vi "Tri. Flow Model (SubVI).vi"(6 "Offset":dbl, 7 "T_Flow Start (s)":dbl, 8 "T_Ejection Period (s)":dbl, 9 "Pressure (mmHg)":waveform(dbl), 10 "T_Flow Peak (s)":dbl, 11 "Flow Amp.":dbl) -> (3 "Triangular  Model Flow":waveform(dbl))   [LabVIEW 2017]
uses:
  <vilib>/Analysis/NI_AALBase.lvlib
  <vilib>/Analysis/1siggen.llb/Ramp Pattern by Samples.vi
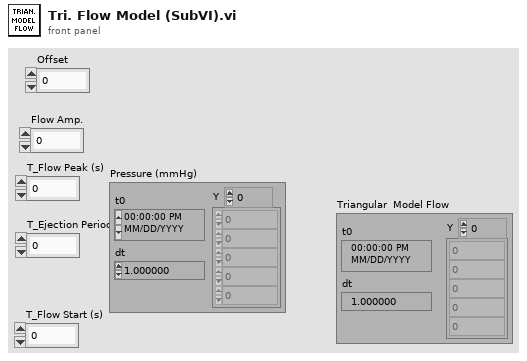
[diagram p1: front panel]
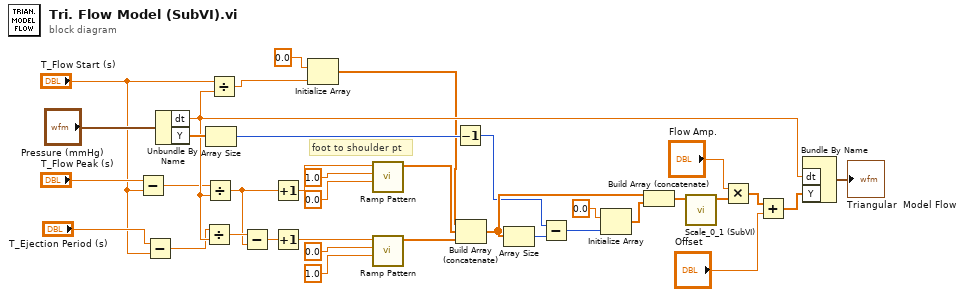
[diagram p0: block diagram]
diagram:
  # "foot to shoulder pt"
  n1 = Subtract(x="T_Flow Peak (s)", y="T_Flow Start (s)") -> (x-y=w4:dbl)
  n2 = Subtract(x="T_Ejection Period (s)", y="T_Flow Start (s)") -> (x-y=w1:dbl)
  n3 = Unbundle By Name("Pressure (mmHg)") -> ("dt"=w13:dbl, "Y"=w17:dbl[])
  n4 = Divide(x=w1, y=w13) -> (x/y=w36:dbl)
  n5 = Divide(x=w4, y=w13) -> (x/y=w21:dbl)
  n6 = Array Size(array=w17) -> (size(s)=w22:i32)
  n7 = Divide(x="T_Flow Start (s)", y=w13) -> (x/y=w10:dbl)
  n8 = Subtract(x=w36, y=w21) -> (x-y=w34:dbl)
  n9 = Increment(x=w21) -> (x+1=w33:dbl)
  n10 = Increment(x=w34) -> (x+1=w35:dbl)
  n11 = Initialize Array(0.0 ("element"), w10) -> (w11:dbl[])
  n12 = call-poly <vilib>:"Ramp Pattern.vi"("start"=0.0, "end"=1.0, "samples"=w33) -> ("Ramp Pattern"=w32:dbl[])  [unwired: 7 in, 1 out]
  n13 = call-poly <vilib>:"Ramp Pattern.vi"("start"=1.0, "end"=0.0, "samples"=w35) -> ("Ramp Pattern"=w20:dbl[])  [unwired: 7 in, 1 out]
  n14 = Decrement(x=w22) -> (x-1=w19:i32)
  n15 = Build Array (concatenate)(w11, w32, w20) -> (w23:dbl[])
  n16 = Array Size(array=w23) -> (size(s)=w27:i32)
  n17 = Subtract(x=w19, y=w27) -> (x-y=w26:i32)
  n18 = Initialize Array(0.0 ("element"), w26) -> (w24:dbl[])
  n19 = Build Array (concatenate)(w23, w24) -> (w14:dbl[])
  n20 = call "Scale_0_1 (SubVI).vi"("BLine D"=w14) -> ("Array"=w15:dbl[])  [unwired: 10 in]
  n21 = Multiply(x="Flow Amp.", y=w15) -> (x*y=w9:dbl[])
  n22 = Add(x=w9, y="Offset") -> (x+y=w8:dbl[])
  n23 = Bundle By Name("dt"=w13, "Y"=w8) -> (→"Triangular  Model Flow":waveform(dbl))  [unwired: 1 in]
